vi "Process Outgoing Frames.vi"(8 "error in (no error)":errorcluster, 9 "timeout ms":i32=100, 11 "Variables":T1={"Process Ref"=refnum, "Comm Ref"=refnum, "Data Refs"={"ProtectionsAndCounters.Ref"=refnum, "Signals.Ref"=refnum, "Status.Ref"=refnum, "Overrides"=refnum, "IncomingSignals.Ref"=refnum, "CtrandProtctnVld.Ref"=refnum, "RcvTime.Ref"=refnum, "TimeDiff.Ref"=refnum, "IncomingProtCtr.Ref"=refnum}, "Settings"={"Name"="", "Priority"=0, "XNET Settings"={"Database"="", "Cluster"="", "Port"="", "Baud rate [Bd]"=0, "Termination"=0, "CAN I/O Mode"=0, "FD Baud rate [Bd]"=500000, "Priority"=100, "Use Legacy"=FALSE, "FD ISO Mode"=0}, "FPGA Session"=0, "Outgoing CAN Session"="", "Outgoing Frame Count"=0, "Outgoing Frames"=[], "Incoming CAN Session"="", "Incoming Frame Count"=0, "Incoming Frames"=[], "Incoming Values"={"Signal Values"=[], "Signal Invalid Values"=[], "ProtCtr Sig Values"=[], "Timestamps"=[], "Time Differences"=[], "IDs"=[]}, "985x Settings"={"Enable"=FALSE, "FPGA Refnum"=refnum, "Channel Number"=0}}, "Stream Refs"={"Addon"="", "Port"="", "Filter Ref"=refnum, "Default Filter"={"ID Filters"=[], "Direction Filter"=enum."Tx/Rx", "Type Filter"=enum."All"}, "Port Settings"={"Mode"=0, "Baud Rate"=0, "Termination"=0, "FD ISO Mode"=0, "FD Baud Rate"=0}}} {"Stream Refs"."Port Settings"."FD ISO Mode" items=["ISO", "Non ISO", "ISO Legacy"]; "Stream Refs"."Port Settings"."Termination" items=["Off", "On"]; "Stream Refs"."Port Settings"."Mode" items=["CAN 2.0", "CAN FD", "CAN FD+BRS"]; "Settings"."XNET Settings"."FD ISO Mode" items=["ISO", "Non ISO", "ISO Legacy"]; "Settings"."XNET Settings"."CAN I/O Mode" items=["CAN 2.0", "CAN FD", "CAN FD+BRS"]; "Settings"."XNET Settings"."Termination" items=["Off", "On"]}) -> (0 "error out":errorcluster, 3 "Variables out":T1={"Process Ref"=refnum, "Comm Ref"=refnum, "Data Refs"={"ProtectionsAndCounters.Ref"=refnum, "Signals.Ref"=refnum, "Status.Ref"=refnum, "Overrides"=refnum, "IncomingSignals.Ref"=refnum, "CtrandProtctnVld.Ref"=refnum, "RcvTime.Ref"=refnum, "TimeDiff.Ref"=refnum, "IncomingProtCtr.Ref"=refnum}, "Settings"={"Name"="", "Priority"=0, "XNET Settings"={"Database"="", "Cluster"="", "Port"="", "Baud rate [Bd]"=0, "Termination"=0, "CAN I/O Mode"=0, "FD Baud rate [Bd]"=500000, "Priority"=100, "Use Legacy"=FALSE, "FD ISO Mode"=0}, "FPGA Session"=0, "Outgoing CAN Session"="", "Outgoing Frame Count"=0, "Outgoing Frames"=[], "Incoming CAN Session"="", "Incoming Frame Count"=0, "Incoming Frames"=[], "Incoming Values"={"Signal Values"=[], "Signal Invalid Values"=[], "ProtCtr Sig Values"=[], "Timestamps"=[], "Time Differences"=[], "IDs"=[]}, "985x Settings"={"Enable"=FALSE, "FPGA Refnum"=refnum, "Channel Number"=0}}, "Stream Refs"={"Addon"="", "Port"="", "Filter Ref"=refnum, "Default Filter"={"ID Filters"=[], "Direction Filter"=enum."Tx/Rx", "Type Filter"=enum."All"}, "Port Settings"={"Mode"=0, "Baud Rate"=0, "Termination"=0, "FD ISO Mode"=0, "FD Baud Rate"=0}}} {"Stream Refs"."Port Settings"."FD ISO Mode" items=["ISO", "Non ISO", "ISO Legacy"]; "Stream Refs"."Port Settings"."Termination" items=["Off", "On"]; "Stream Refs"."Port Settings"."Mode" items=["CAN 2.0", "CAN FD", "CAN FD+BRS"]; "Settings"."XNET Settings"."FD ISO Mode" items=["ISO", "Non ISO", "ISO Legacy"]; "Settings"."XNET Settings"."CAN I/O Mode" items=["CAN 2.0", "CAN FD", "CAN FD+BRS"]; "Settings"."XNET Settings"."Termination" items=["Off", "On"]})   [LabVIEW 2020, in "Protection and Counter Addon Engine.lvlib"]
uses:
  Protection and Counter Addon Engine.lvlib
  Types/RT Async Engine Variables.ctl
  <vilib>/NI/NIVS Inline Async API/_VS Inline Async API/Process/Process.lvclass
  <vilib>/NI/NI VeriStand Addon Network Comm/Engine/VeriStand Comm.lvclass
  Types/RT Data References.ctl
  <vilib>/NI/NIVS Inline Async API/_Data Access Engine/Data Access Engine/Types/Write.DVR.ctl
  <vilib>/NI/NIVS Inline Async API/_Data Access Engine/Access Type Classes/Write/Write.lvclass
  <vilib>/NI/NIVS Inline Async API/_Data Access Engine/Data Access Engine/Types/Read.DVR.ctl
  <vilib>/NI/NIVS Inline Async API/_Data Access Engine/Access Type Classes/Read/Read.lvclass
  Types/RT Async Engine Settings.ctl
  Addon Shared/Types/XNET Settings.ctl
  SubModules/Frame-Protection-Support/Source/Engine/Types/RT Frame Settings.ctl
  SubModules/Frame-Protection-Support/Source/Shared/Types/Exported Frame Type.ctl
  SubModules/Frame-Protection-Support/Source/Engine/Types/RT Protection Configuration.ctl
  SubModules/Frame-Protection-Support/Source/Shared/Types/Protection Type.ctl
  SubModules/Frame-Protection-Support/Source/Shared/Types/XNET Signal Configuration.ctl
  SubModules/Frame-Protection-Support/Source/Shared/Types/Exported Counter Settings.ctl
  SubModules/Frame-Protection-Support/Source/Shared/Types/Exported Event Trigger Type.ctl
  SubModules/Frame-Protection-Support/Source/Engine/Types/RT Frame Incoming Values.ctl
  SubModules/985x-Support/Source/Addon Engine/Types/985x Settings.ctl
  SubModules/985x-Support/Source/Addon Engine/Types/FPGA Refnum.ctl
  SubModules/CAN-Streaming-Support/Source/Addon/Addon Engine/Types/Engine Stream Refs.ctl
  SubModules/CAN-Streaming-Support/Source/Addon/Addon Shared/Types/Direction Filter.ctl
  SubModules/CAN-Streaming-Support/Source/Addon/Addon Shared/Types/Type Filter.ctl
  SubModules/CAN-Streaming-Support/Source/Addon/Addon Shared/Types/Filter Parameters.ctl
  SubModules/CAN-Streaming-Support/Source/Addon/Addon Engine/Types/Engine Stream Port Settings.ctl
  <vilib>/NI/NIVS Inline Async API/_Data Access Engine/Access Type Classes/Read/Read.lvclass/Read.ctl
  <vilib>/NI/NIVS Inline Async API/_Data Access Engine/Access Type Classes/Write/Write.lvclass/Write.ctl
  <vilib>/NI/NIVS Inline Async API/_Data Access Engine/Data Access Engine/Methods/Write.Data.vi
  <vilib>/NI/NIVS Inline Async API/_Data Access Engine/Access Type Classes/Write/Write.ProcessData.vi
  <vilib>/NI/NIVS Inline Async API/_Data Access Engine/Data Access Engine/Methods/Read.Data.Detect.vi
  <vilib>/NI/NIVS Inline Async API/_Data Access Engine/Data Access Engine/Methods/Read.Data.vi
  SubModules/Frame-Protection-Support/Source/Engine/SubVIs/Determine Transmit.vi
  SubModules/Frame-Protection-Support/Source/Engine/SubVIs/Update Counter Signals.vi
  SubModules/Frame-Protection-Support/Source/Engine/SubVIs/Get Frame Data.vi
  SubModules/Frame-Protection-Support/Source/Engine/SubVIs/Convert EU Data to XNET Frame.vi
  SubModules/Frame-Protection-Support/Source/Engine/SubVIs/Update Protection Signals.vi
  SubModules/Frame-Protection-Support/Source/Engine/SubVIs/Determine Disabled.vi
  <vilib>/NI/NIVS Inline Async API/_Data Access Engine/Data Access Engine/Methods/Write.Data.Commit.vi
  <vilib>/NI/NIVS Inline Async API/_Data Access Engine/Access Type Classes/Write/Write.Buffer.vi
  <vilib>/NI/NIVS Inline Async API/_Data Access Engine/Access Type Classes/Write/Write.Commit.vi
  <vilib>/NI/NIVS Inline Async API/_Data Access Engine/Access Type Classes/Read/Read.ProcessData.Detect.vi
  <vilib>/NI/NIVS Inline Async API/_Data Access Engine/Access Type Classes/Read/Read.ProcessData.vi
  SubModules/Frame-Protection-Support/Source/Engine/SubVIs/Determine Transmission.vi
  SubModules/Frame-Protection-Support/Source/Engine/SubVIs/Determine Periodic.vi
  SubModules/Frame-Protection-Support/Source/Engine/SubVIs/Set Counter Signal.vi
  SubModules/Frame-Protection-Support/Source/Engine/SubVIs/Calculate Counter Value.vi
  SubModules/Frame-Protection-Support/Source/Engine/SubVIs/Set Protection Signal.vi
  SubModules/Frame-Protection-Support/Source/Engine/SubVIs/Calculate Protection Value.vi
  <vilib>/NI/NIVS Inline Async API/_Data Access Engine/Data Access Engine/Methods/Write.Data.Buffer.vi
  SubModules/Frame-Protection-Support/Source/Engine/SubVIs/Get Protection Signals.vi
  <vilib>/xnet/xnet.llb/XNET Convert.vi
  <vilib>/xnet/xnet.llb/XNET Convert (Signal to Frame Raw).vi
  <vilib>/xnet/xnet.llb/XNET Convert (Signal to Frame CAN).vi
  <vilib>/xnet/xnet.llb/XNET Write (Frame CAN).vi
  <vilib>/NI/NIVS Inline Async API/_Data Access Engine/Data Access Engine/Data Access Engine.lvclass
  SubModules/Frame-Protection-Support/Source/Engine/Protection and Counter Support Engine.lvlib
  SubModules/985x-Support/Source/Addon Engine/985x Support Addon Engine.lvlib
  SubModules/Frame-Protection-Support/Source/Shared/Protection and Counter Support Shared.lvlib
  SubModules/CAN-Streaming-Support/Source/Addon/Addon Shared/CAN Stream Support Shared.lvlib
  SubModules/CAN-Streaming-Support/Source/Addon/Addon Engine/CAN Stream Support Engine.lvlib
  Addon Shared/Protection and Counter Addon Shared.lvlib
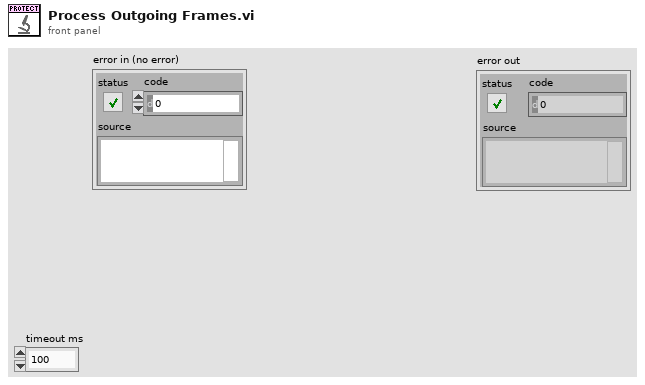
[diagram p1: front panel]
types:
  T1 = typedef "Protection and Counter Addon Engine.lvlib/RT Async Engine Variables.ctl" = cluster{"Process Ref":refnum<class "Process.lvclass">, "Comm Ref":refnum<class "VeriStand Comm.lvclass">, "Data Refs":T2, "Settings":T5, "Stream Refs":T17}
  T2 = typedef "Protection and Counter Addon Engine.lvlib/RT Data References.ctl" = cluster{"ProtectionsAndCounters.Ref":T3, "Signals.Ref":T4, "Status.Ref":T3, "Overrides":T4, "IncomingSignals.Ref":T3, "CtrandProtctnVld.Ref":T3, "RcvTime.Ref":T3, "TimeDiff.Ref":T3, "IncomingProtCtr.Ref":T3}
  T3 = typedef "Data Access Engine.lvlib/Data Access Engine.lvclass/Write.DVR.ctl" = refnum<data-value>
  T4 = typedef "Data Access Engine.lvlib/Data Access Engine.lvclass/Read.DVR.ctl" = refnum<data-value>
  T5 = typedef "Protection and Counter Addon Engine.lvlib/RT Async Engine Settings.ctl" = cluster{"Name":string, "Priority":i32, "XNET Settings":T6, "FPGA Session":u32, "Outgoing CAN Session":refnum<k21>, "Outgoing Frame Count":i32, "Outgoing Frames":T7[], "Incoming CAN Session":refnum<k21>, "Incoming Frame Count":i32, "Incoming Frames":T7[], "Incoming Values":T14, "985x Settings":T15}
  T6 = typedef "Protection and Counter Addon Shared.lvlib/XNET Settings.ctl" = cluster{"Database":refnum<k21>, "Cluster":refnum<k21>, "Port":string, "Baud rate [Bd]":u64, "Termination":u32, "CAN I/O Mode":u32, "FD Baud rate [Bd]":u64, "Priority":i32, "Use Legacy":bool, "FD ISO Mode":u32}
  T7 = typedef "Protection and Counter Support Engine.lvlib/RT Frame Settings.ctl" = cluster{"Type":T8, "Frame ID":u32, "Payload Length":u32, "VS Offset":i32, "VS Length":i32, "Frame Conversion":refnum<k21>, "Frame.Data":dbl[], "Generation Period":u32, "Time Since Last Generation":u32, "Generation Iterations":u32, "Generation Counter":u32, "Has Protection?":bool, "Protection Configurations":T9[], "Has Counter?":bool, "Counter Configurations":T12[], "Has Disable?":bool, "Disable VS Index":i32, "Transmit Trigger":T13, "Trigger VS Index":i32}
  T8 = typedef "Protection and Counter Support Shared.lvlib/Exported Frame Type.ctl" = enum16{"Periodic", "Event", "Periodic/Event"}
  T9 = typedef "Protection and Counter Support Engine.lvlib/RT Protection Configuration.ctl" = cluster{"Protection Frame Index":i32, "Protection Type":T10, "Data Indeces":i32[], "Data Array":dbl[], "Check Sum Conversion":refnum<k21>, "CRC Channels":T11[], "Protection VS Index":i32, "Counter Data Index":i32, "Override Index":i32, "Override Value Index":i32}
  T10 = typedef "Protection and Counter Support Shared.lvlib/Protection Type.ctl" = enum16{"Arb ID + Bytes Checksum with Inversion", "Arb ID + Bytes CRC with Inversion", "Reversed Raw Signal Checksum with Inversion", "Concatenated Two's Compliment"}
  T11 = typedef "Protection and Counter Support Shared.lvlib/XNET Signal Configuration.ctl" = cluster{"Start Bit":i32, "Name":string, "Number of bits":i32, "Scale":dbl, "Offset":dbl, "Data Type":u32, "Counter":bool}
  T12 = typedef "Protection and Counter Support Shared.lvlib/Exported Counter Settings.ctl" = cluster{"Frame Index":i32, "Max Count":dbl, "VS Index":i32, "Bit Length":i64, "Override Index":i32, "Override Value Index":i32}
  T13 = typedef "Protection and Counter Support Shared.lvlib/Exported Event Trigger Type.ctl" = enum16{"Channel value change", "Trigger channel (not zero)", "Channel value change or trigger channel (not zero)", "Trigger channel (any value change)", "Channel value change or trigger channel (any value change)"}
  T14 = typedef "Protection and Counter Support Engine.lvlib/RT Frame Incoming Values.ctl" = cluster{"Signal Values":dbl[], "Signal Invalid Values":dbl[], "ProtCtr Sig Values":dbl[], "Timestamps":timestamp[], "Time Differences":dbl[], "IDs":u32[]}
  T15 = typedef "985x Support Addon Engine.lvlib/985x Settings.ctl" = cluster{"Enable":bool, "FPGA Refnum":T16, "Channel Number":u32}
  T16 = typedef "985x Support Addon Engine.lvlib/FPGA Refnum.ctl" = refnum<k20>
  T17 = typedef "CAN Stream Support Engine.lvlib/Engine Stream Refs.ctl" = cluster{"Addon":string, "Port":refnum<k21>, "Filter Ref":refnum<data-value>, "Default Filter":T18, "Port Settings":T21}
  T18 = typedef "CAN Stream Support Shared.lvlib/Filter Parameters.ctl" = cluster{"ID Filters":u32[], "Direction Filter":T19, "Type Filter":T20}
  T19 = typedef "CAN Stream Support Shared.lvlib/Direction Filter.ctl" = enum16{"Tx/Rx", "Rx", "Tx"}
  T20 = typedef "CAN Stream Support Shared.lvlib/Type Filter.ctl" = enum16{"All", "CAN Data", "CAN Remote", "CAN Bus Error", "CAN 2.0 Data", "CAN FD Data", "CAN FD+BRS Data", "J1939 Data", "Delay", "Log Trigger", "Start Trigger"}
  T21 = typedef "CAN Stream Support Engine.lvlib/Engine Stream Port Settings.ctl" = cluster{"Mode":u32, "Baud Rate":u64, "Termination":u32, "FD ISO Mode":u32, "FD Baud Rate":u64}
  T22 = typedef "XNET Frame CAN.ctl" = cluster{"timestamp":timestamp, "payload":u8[], "identifier":u32, "type":T23, "extended?":bool, "echo?":bool}
  T23 = typedef "XNET Frame Type CAN.ctl" = u8
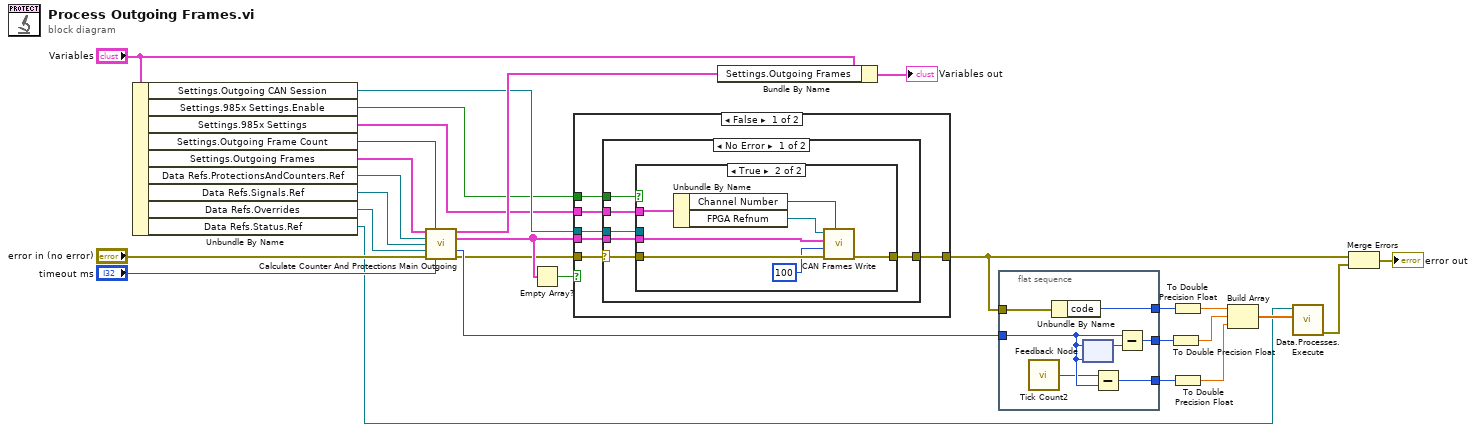
[diagram p0: block diagram]
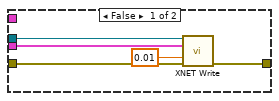
[diagram p2: hidden frame]
diagram:
  n1 = Unbundle By Name("Variables") -> ("Settings.Outgoing CAN Session"=w12:refnum<k21>, "Settings.985x Settings.Enable"=w2:bool, "Settings.985x Settings"=w1:T15, "Settings.Outgoing Frame Count"=w26:i32, "Settings.Outgoing Frames"=w9:T7[], "Data Refs.ProtectionsAndCounters.Ref"=w4:T3, "Data Refs.Signals.Ref"=w5:T4, "Data Refs.Overrides"=w3:T4, "Data Refs.Status.Ref"=w6:T3)
  n2 = call "Calculate Counter And Protections Main Outgoing.vi"("Frames in"=w9, "Frame Count"=w26, "Protections"=w4, "Signals"=w5, "Overrides"=w3, "error in (no error)"="error in (no error)", "timeout ms"="timeout ms") -> ("Frames out"=w16:T7[], "Frames"=w15:T22[], "Tick Count(uSec)"=w24:u32, "error out"=w11:errorcluster)  [unwired: 5 in]
  n3 = Empty Array?(array=w15) -> (empty?=w14:bool)
  n4 = case shown="False" w14 {
    tunnel: w11 -> [w34 w54]
    tunnel: [w33 w54] -> w10
    tunnel: w12 -> [w32 _]
    tunnel: w15 -> [w31 _]
    tunnel: w2 -> [w30 _]
    tunnel: w1 -> [w29 _]
    frame False {
      n5 = case shown="No Error" w34 {
        selector: w34 -> [w37 w53]
        tunnel: w31 -> [w40 _]
        tunnel: [w39 w53] -> w33
        tunnel: w32 -> [w38 _]
        tunnel: w30 -> [w36 _]
        tunnel: w29 -> [w35 _]
        frame No Error {
          n6 = case shown="True" w36 {
            tunnel: w40 -> [w45 w51]
            tunnel: [w44 w49] -> w39
            tunnel: w38 -> [w43 _]
            tunnel: w37 -> [w42 w50]
            tunnel: w35 -> [_ w52]
            frame False {
              n7 = call-poly <vilib>:"XNET Write.vi"("session in"=w43, "data"=w45, "timeout (10)"=0.01, "error in (no error)"=w42) -> ("error out"=w44:errorcluster)  [unwired: 10 in, 1 out]
            }
            frame True {
              n8 = Unbundle By Name(w52) -> ("Channel Number"=w48:u32, "FPGA Refnum"=w47:T16)
              n9 = call "CAN Frames Write.vi"("Channel Number"=w48, "error in (no error)"=w50, "Timeout (ms)"=100, "Frames"=w51, "FPGA Refnum"=w47) -> ("error out"=w49:errorcluster)  [unwired: 6 in]
            }
          }
        }
        frame Error {
        }
      }
    }
    frame True {
    }
  }
  n10 = Bundle By Name(cluster="Variables", "Settings.Outgoing Frames"=w16) -> (→"Variables out":T1)
  n11 = flat-sequence {
    tunnel: w24 -> [w61]
    tunnel: [w60] -> w23
    tunnel: [w59] -> w20
    tunnel: w10 -> [w56]
    tunnel: [w55] -> w13
    frame #0 {
      n12 = call "Tick Count2"() -> ("Tick Count(uSec)"=w58:u32)
      n13 = Unbundle By Name(w56) -> ("code"=w55:i32)
      n14 = feedback #1(w61) -> (w57:u32)
      n15 = feedback-in #1(w61) -> ()
      n16 = Subtract(x=w58, y=w61) -> (x-y=w59:u32)
      n17 = Subtract(x=w61, y=w57) -> (x-y=w60:u32)
    }
  }
  n18 = To Double Precision Float(number=w23) -> (double precision float=w18:dbl)
  n19 = To Double Precision Float(number=w13) -> (double precision float=w19:dbl)
  n20 = To Double Precision Float(number=w20) -> (double precision float=w17:dbl)
  n21 = Build Array(w19, w18, w17) -> (w22:dbl[])
  n22 = call-poly <vilib>:"Data.Processes.Execute.vi"("Values"=w22, "Ref"=w6) -> ("error out"=w21:errorcluster)  [unwired: 9 in]
  n23 = Merge Errors(w10, w21) -> (→"error out":errorcluster)
